vi "Read PM Sensor Channel.vi"(0 "VISA session":refnum<visa-resource-name>="PM1", 1 "Measuring Function (0: Single)":i32(ring) items=["Single", "Single Relative", "Difference", "Difference Relative", "Ratio", "Ratio Relative"], 3 "Measurement Speed":i32, 5 "Channel (0: A)":i32(ring) items=["A", "B"], 7 "State (T: On)":bool, 9 "Input parameters":T1={"Channel (1)"=1, "Avg Count"=4, "Correction Frequency"=50000000.0, "Timeout"=10000, "Reset Device"=FALSE, "ID Query"=FALSE, "Resource Name"="PM1", "Ref Level (dB)"=20.0} {"Ref Level (dB)" format="%^.2e"; "Correction Frequency" format="%.2p"}, 11 "error in":errorcluster, 12 "Pwr Mtr Cal":bool=TRUE, 14 "Route Names":string[](array[string])) -> (4 "dup VISA session":refnum<visa-resource-name>, 6 "dBm":dbl format="%.5f", 15 "error out":errorcluster)   [LabVIEW 2015]
doc: "This VI runs one sensor measurement.\n- Open session to sensor specified by Resource Name\n- Sets correct frequency\n- Initialize acqusistion, wait specified time for measurement and reads it."
panel:
  in  "Window (1)":i32=1
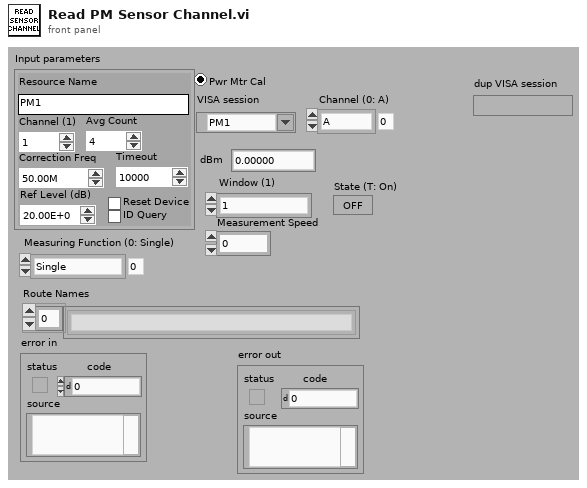
[diagram p1: front panel]
types:
  T1 = cluster{"Channel (1)":i32, "Avg Count":i32, "Correction Frequency":dbl, "Timeout":i32, "Reset Device":bool, "ID Query":bool, "Resource Name":string, "Ref Level (dB)":dbl}
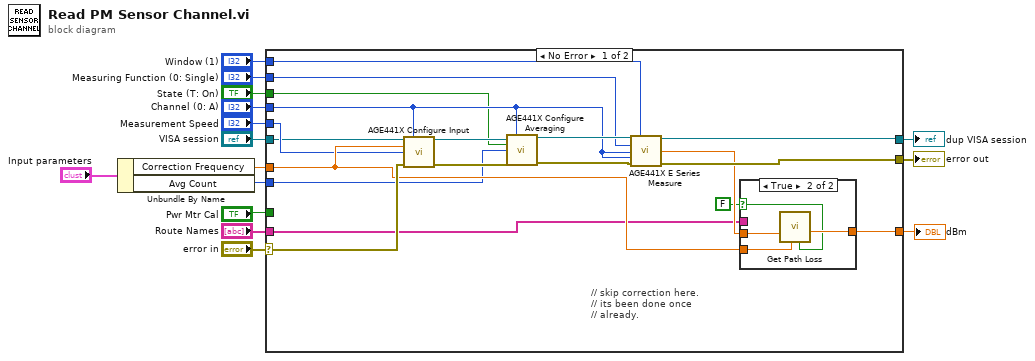
[diagram p0: block diagram]
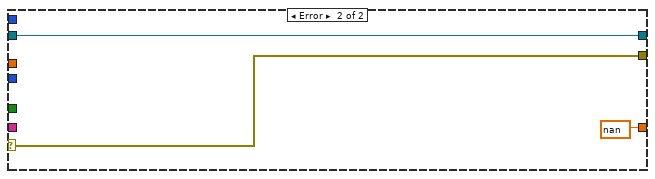
[diagram p3: hidden frame]
diagram:
  n1 = Unbundle By Name("Input parameters") -> ("Correction Frequency"=w11:dbl, "Avg Count"=w10:i32)
  n2 = case shown="No Error" "error in" {
    selector: "error in" -> [w34 w42]
    tunnel: [w33 w42] -> w14
    tunnel: "Channel (0: A)" -> [w20 _]
    tunnel: w11 -> [w31 _]
    tunnel: w10 -> [w23 _]
    tunnel: "Measurement Speed" -> [w27 _]
    tunnel: "VISA session" -> [w26 w41]
    tunnel: [w25 w41] -> w7
    tunnel: "Window (1)" -> [w22 _]
    tunnel: "Measuring Function (0: Single)" -> [w21 _]
    tunnel: "State (T: On)" -> [w19 _]
    tunnel: [w18 nan ("Adjusted Power Level")] -> w3
    tunnel: "Pwr Mtr Cal" -> [_ _]
    tunnel: "Route Names" -> [w17 _]
    frame No Error {
      # "// skip correction here.\n// its been done once\n// already."
      n3 = call <instrlib>:"AGE441X Configure Input.vi"("VISA session"=w26, "Channel (0: A)"=w20, "Frequency (50.00 E+6)"=w31, "Measurement Speed (0: Normal)"=w27, "error in (no error)"=w34) -> ("dup VISA session"=w28:refnum<visa-resource-name>, "error out"=w30:errorcluster)  [unwired: 9 in]
      n4 = call <instrlib>:"AGE441X Configure Averaging.vi"("VISA session"=w28, "Channel (0: A)"=w20, "State (T: On)"=w19, "Filter Length (4)"=w23, "error in (no error)"=w30) -> ("dup VISA session"=w24:refnum<visa-resource-name>, "error out"=w29:errorcluster)  [unwired: 9 in]
      n5 = call <instrlib>:"AGE441X E Series Measure.vi"("VISA session"=w24, "Measurement (1)"=w22, "Measuring Function (0: Single)"=w21, "Sensor 1 (0: Channel A)"=w20, "Sensor 2 (0: Channel A)"=w20, "error in (no error)"=w29) -> ("dup VISA session"=w25:refnum<visa-resource-name>, "Measured Value"=w32:dbl, "error out"=w33:errorcluster)  [unwired: 7 in]
      n6 = case shown="True" FALSE {
        selector: FALSE -> [_ w36]
        tunnel: w31 -> [_ w39]
        tunnel: w32 -> [w35 w38]
        tunnel: [w35 w37] -> w18
        tunnel: w17 -> [_ _]
        frame False {
        }
        frame True {
          n7 = call "Get Path Loss.vi"("Calibration Enabled"=w36, "Frequency"=w39, "Power Level"=w38) -> ("Adjusted Power Level"=w37:dbl)  [unwired: 4 in, 4 out]
        }
      }
    }
    frame Error {
    }
  }
  "error out" <- w14
  "dup VISA session" <- w7
  "dBm" <- w3
